vi "Cargo Angle TeleOp.vi"(11 "Cluster":cluster{"Cluster":T1}) -> ()   [LabVIEW 2018]
uses:
  Controller Values.ctl
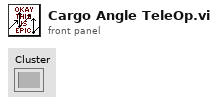
[diagram p1: front panel]
types:
  T1 = typedef "Controller Values.ctl" = cluster{"Left Joystick Axes ":dbl[], "Right Joystick Axes":dbl[], "Left Joystick Buttons":bool[], "Right Joystick Buttons":bool[], "DDR Buttons":bool[], "XBox Axes":dbl[], "XBox Buttons":bool[], "XBox POVs":i16[]}
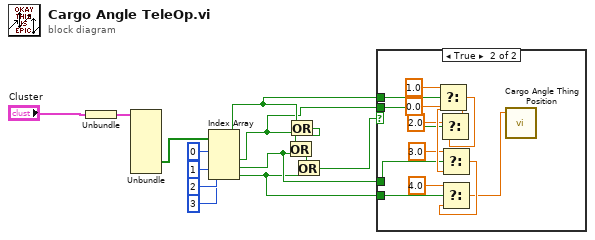
[diagram p0: block diagram]
diagram:
  n1 = Unbundle("Cluster") -> ("Cluster"=w13:T1)
  n2 = Unbundle(w13) -> ("XBox Buttons"=w12:bool[])  [unwired: 7 out]
  n3 = Index Array(array=w12, index #1=0 ("index"), index #2=1 ("index"), index #3=2 ("index"), index #4=3 ("index")) -> (element #1=w4:bool, element #2=w3:bool, element #3=w2:bool, element #4=w1:bool)
  n4 = Or(x=w4, y=w3) -> (x .or. y?=w7:bool)
  n5 = Or(x=w7, y=w2) -> (x .or. y?=w6:bool)
  n6 = Or(x=w6, y=w1) -> (x .or. y?=w5:bool)
  n7 = case shown="True" w5 {
    tunnel: w4 -> [_ w23]
    tunnel: w3 -> [_ w22]
    tunnel: w2 -> [_ w21]
    tunnel: w1 -> [_ w20]
    frame False {
    }
    frame True {
      n8 = Select(t=1.0, s=w23, f=0.0) -> (s? t:f=w27:dbl)
      n9 = Select(t=2.0, s=w22, f=w27) -> (s? t:f=w26:dbl)
      n10 = Select(t=3.0, s=w21, f=w26) -> (s? t:f=w25:dbl)
      n11 = Select(t=4.0, s=w20, f=w25) -> (s? t:f=w24:dbl)
      n12 = call "Cargo Angle Thing Position.vi"("Setpoint"=w24) -> ()  [unwired: 10 in, 1 out]
    }
  }
